vi "camera_diag.vi"() -> ()   [LabVIEW 2013]
uses:
  Program Files/Andor SOLIS/Drivers 32bit/Examples/LabVIEW/System Files/user.lib/atmcd32d.llb/AcquisitionMode_mode typedef.ctl
  Program Files/Andor SOLIS/Drivers 32bit/Examples/LabVIEW/System Files/user.lib/atmcd32d.llb/ReadMode_mode typedef.ctl
  Program Files/Andor SOLIS/Drivers 32bit/Examples/LabVIEW/System Files/user.lib/atmcd32d.llb/Error Code Enum typedef.ctl
panel:
  out "Status":u32
  out "DLL error code 3":u32
  out "output array":i32[][](graph)
  in  "FT Mode":enum16{"OFF", "ON"}(ring)
  out "DLL error code 2":u32
  out "DLL error code":u32
  out "SetKinError":u32
  out "Calculated Exposure Value":sgl format="%.2f"
  out "Calculated Kinetic Value":sgl format="%.2f"
  in  "Exposure Time (secs)":sgl format="%.2f"
  in  "Number of Kinetics":i32
  in  "Kinetic Cycle Time (s)":sgl format="%.2f"
  in  "Trigger":u32(ring) items=["Internal", "External"]
  in  "mode":T1=enum."Single Scan"
  in  "shutdown":bool
  in  "GO":bool
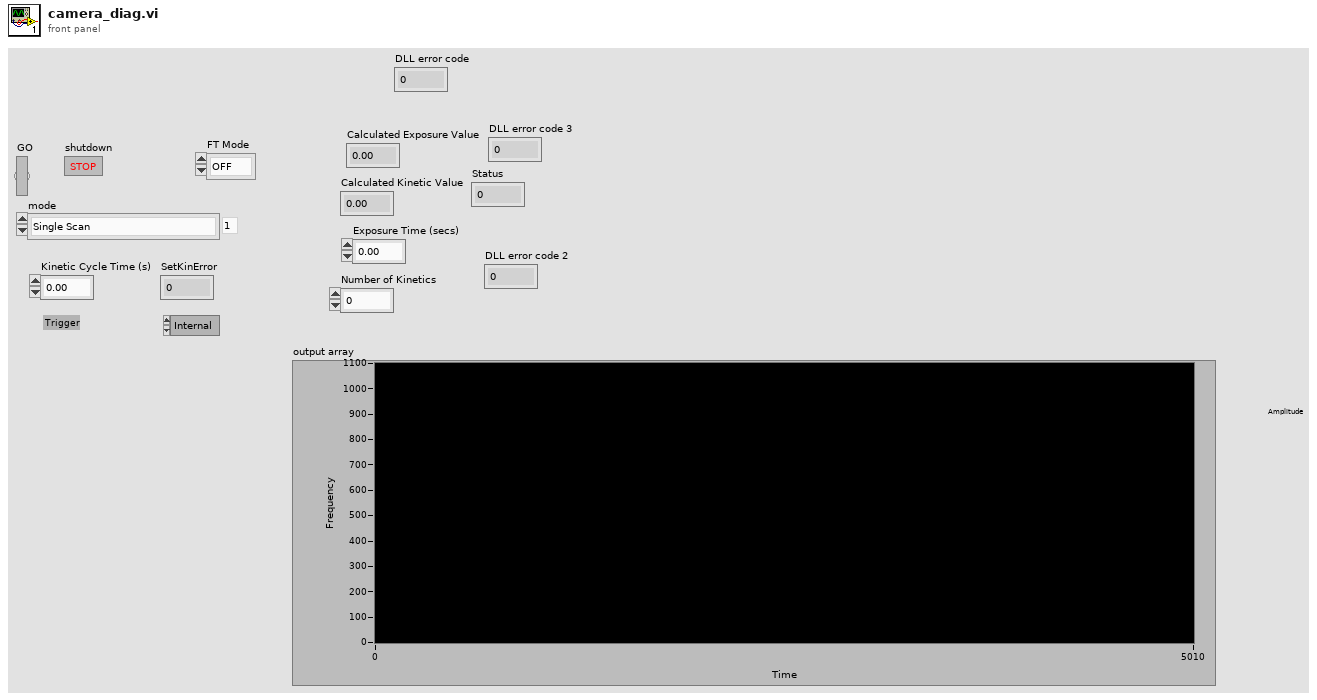
[diagram p1: front panel]
types:
  T1 = typedef "AcquisitionMode_mode typedef.ctl" = enum16{"Reserved (0)", "Single Scan", "Accumulate", "Kinetics", "Fast Kinetics", "Run Till Abort", "Reserved (6)", "Reserved (7)", "Reserved (8)", "Time Delayed Integration"}
  T2 = typedef "ReadMode_mode typedef.ctl" = enum16{"Full Vertical Binning", "Multi-Track", "Random-Track", "Single-Track", "Image"}
  T3 = typedef "Error Code Enum typedef.ctl" = enum32{"N/A (0)", "DRV_ERROR_CODES", "DRV_SUCCESS", "DRV_VXDNOTINSTALLED", "DRV_ERROR_SCAN", "DRV_ERROR_CHECK_SUM", "DRV_ERROR_FILELOAD", "DRV_UNKNOWN_FUNC", "DRV_ERROR_VXD_INIT", "DRV_ERROR_ADDRESS", "DRV_ERROR_PAGELOCK", "DRV_ERROR_PAGEUNLOCK", "DRV_ERROR_BOARDTEST", "DRV_ERROR_ACK", "DRV_ERROR_UP_FIFO", "DRV_ERROR_PATTERN", "N/A (16)", "DRV_ACQUISITION_ERRORS", "DRV_ACQ_BUFFER", "DRV_ACQ_DOWNFIFO_FULL", "DRV_PROC_UNKONWN_INSTRUCTION", "DRV_ILLEGAL_OP_CODE", "DRV_KINETIC_TIME_NOT_MET", "DRV_ACCUM_TIME_NOT_MET", "DRV_NO_NEW_DATA", "N/A (25)", "DRV_SPOOLERROR", "N/A (27)", "N/A (28)", "N/A (29)", "N/A (30)", "N/A (31)", "N/A (32)", "DRV_TEMPERATURE_CODES", "DRV_TEMPERATURE_OFF", "DRV_TEMPERATURE_NOT_STABILIZED", "DRV_TEMPERATURE_STABILIZED", "DRV_TEMPERATURE_NOT_REACHED", "DRV_TEMPERATURE_OUT_RANGE", "DRV_TEMPERATURE_NOT_SUPPORTED", "DRV_TEMPERATURE_DRIFT", "N/A (41)", "N/A (42)", "N/A (43)", "N/A (44)", "N/A (45)", "N/A (46)", "N/A (47)", "N/A (48)", "DRV_GENERAL_ERRORS", "DRV_INVALID_AUX", "DRV_COF_NOTLOADED", "DRV_FPGAPROG", "DRV_FLEXERROR", "DRV_GPIBERROR", "N/A (55)", "N/A (56)", "N/A (57)", "N/A (58)", "N/A (59)", "N/A (60)", "N/A (61)", "N/A (62)", "N/A (63)", "DRV_DATATYPE", "DRV_DRIVER_ERRORS", "DRV_P1INVALID", "DRV_P2INVALID", "DRV_P3INVALID", "DRV_P4INVALID", "DRV_INIERROR", "DRV_COFERROR", "DRV_ACQUIRING", "DRV_IDLE", "DRV_TEMPCYCLE", "DRV_NOT_INITIALIZED", "DRV_P5INVALID", "DRV_P6INVALID", "DRV_INVALID_MODE", "DRV_INVALID_FILTER", "DRV_I2CERRORS", "DRV_I2CDEVNOTFOUND", "DRV_I2CTIMEOUT", "DRV_P7INVALID", "N/A (84)", "N/A (85)", "N/A (86)", "N/A (87)", "N/A (88)", "N/A (89)", "DRV_IOCERROR", "DRV_VRMVERSIONERROR"}
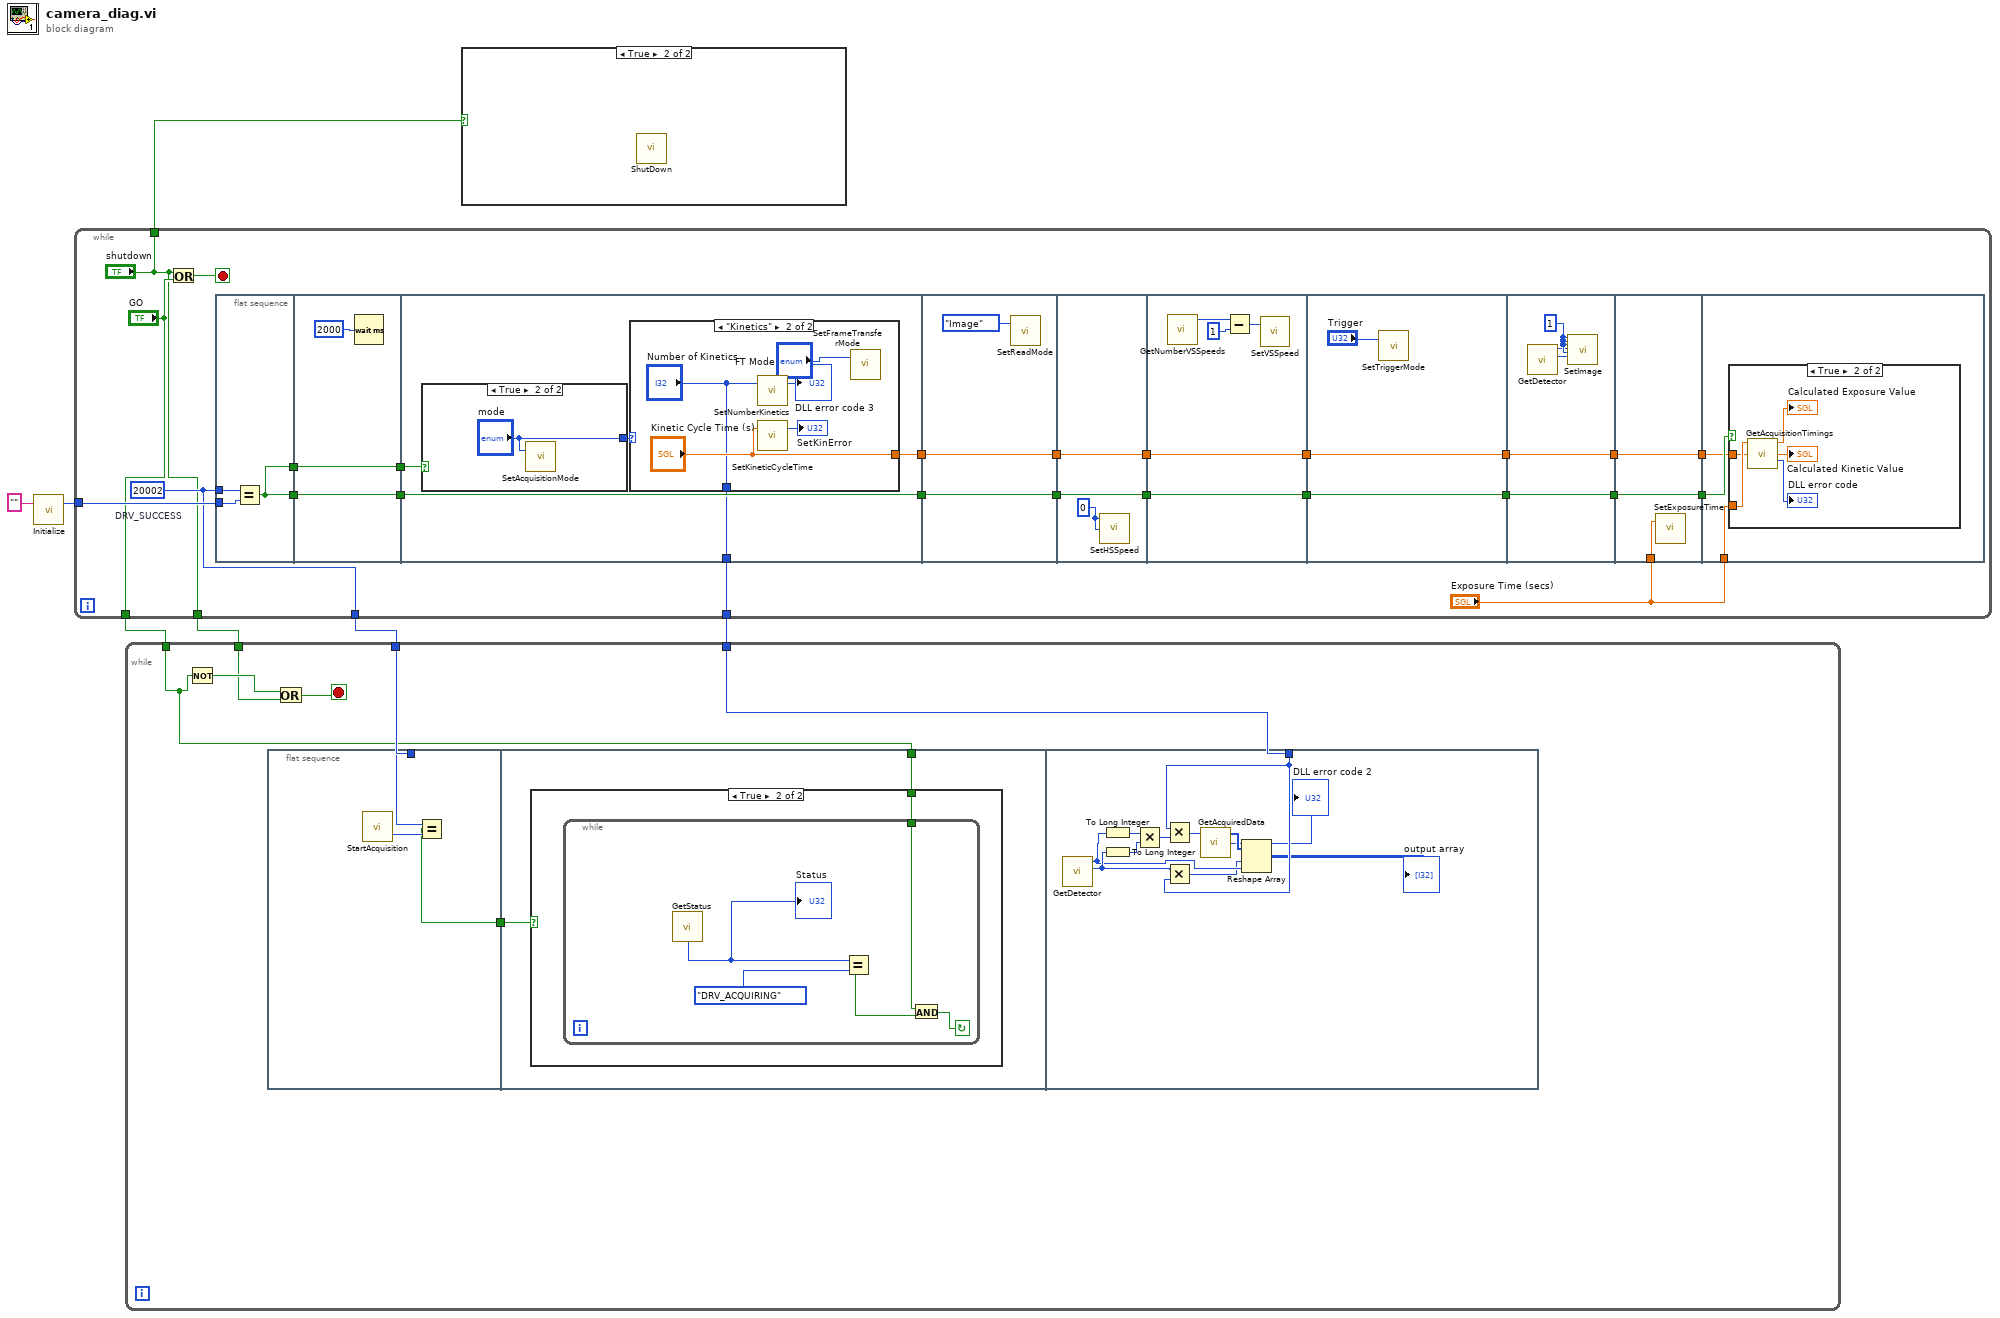
[diagram p0: block diagram]
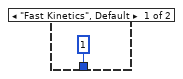
[diagram p4: hidden frame]
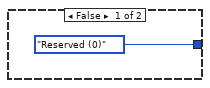
[diagram p5: hidden frame]
diagram:
  n1 = call "Initialize.vi"("directory (\"\")"="" ("directory (\"\")")) -> ("DLL error code"=w6:u32)  [unwired: 1 in, 1 out]
  n2 = while {
    tunnel: w6 -> [w31]
    tunnel: ["GO"] -> w5
    tunnel: [w10] -> w4
    tunnel: [w9] -> w3
    tunnel: ["shutdown"] -> w2
    tunnel: ["shutdown"] -> w1
    stop <- w32 stop-if-true
    w10 = 20002  # DRV_SUCCESS
    n3 = Or(x="shutdown", y="GO") -> (x .or. y?=w32:bool)
    n4 = flat-sequence {
      tunnel: w31 -> [w35]
      tunnel: w10 -> [w34]
      tunnel: [w33] -> w29
      tunnel: [w33] -> w20
      tunnel: [w37] -> w30
      tunnel: w29 -> [w37]
      tunnel: [w36] -> w21
      tunnel: w20 -> [w36]
      tunnel: w30 -> [w43]
      tunnel: [w41] -> w22
      tunnel: w21 -> [w41]
      tunnel: [w40] -> w12
      tunnel: [w39] -> w9
      tunnel: [w53] -> w23
      tunnel: w22 -> [w53]
      tunnel: [w52] -> w13
      tunnel: w12 -> [w52]
      tunnel: [w56] -> w24
      tunnel: w23 -> [w56]
      tunnel: [w55] -> w14
      tunnel: w13 -> [w55]
      tunnel: [w59] -> w25
      tunnel: w24 -> [w59]
      tunnel: [w58] -> w15
      tunnel: w14 -> [w58]
      tunnel: [w64] -> w26
      tunnel: w25 -> [w64]
      tunnel: [w63] -> w16
      tunnel: w15 -> [w63]
      tunnel: [w67] -> w27
      tunnel: w26 -> [w67]
      tunnel: [w66] -> w17
      tunnel: w16 -> [w66]
      tunnel: "Exposure Time (secs)" -> [w73]
      tunnel: [w72] -> w28
      tunnel: w27 -> [w72]
      tunnel: [w71] -> w18
      tunnel: w17 -> [w71]
      tunnel: w28 -> [w76]
      tunnel: "Exposure Time (secs)" -> [w75]
      tunnel: w18 -> [w74]
      frame #0 {
        n5 = Equal?(x=w34, y=w35) -> (x = y?=w33:bool)
      }
      frame #1 {
        n6 = Wait (ms)(milliseconds to wait=u32 2000) -> ()  [unwired: 1 out]
      }
      frame #2 {
        n7 = case shown="True" w43 {
          tunnel: [AcquisitionMode_mode_typedef."Reserved (0)" ("mode") "mode"] -> w42
          frame False {
          }
          frame True {
            n8 = call "SetAcquisitionMode.vi"("mode"="mode") -> ()  [unwired: 1 in, 2 out]
          }
        }
        n9 = case shown="\"Kinetics\"" w42 {
          tunnel: [_ "Kinetic Cycle Time (s)"] -> w40
          tunnel: [1 ("Number of Kinetics") "Number of Kinetics"] -> w39
          frame "Fast Kinetics", Default {
          }
          frame "Kinetics" {
            n10 = call <userlib>:"SetNumberKinetics.vi"("number"="Number of Kinetics") -> ("DLL error code"=→"DLL error code 3":u32)  [unwired: 1 in, 1 out]
            n11 = call <userlib>:"SetKineticCycleTime.vi"("time"="Kinetic Cycle Time (s)") -> ("DLL error code"=→"SetKinError":u32)  [unwired: 1 in, 1 out]
            n12 = call "SetFrameTransferMode.vi"("mode"="FT Mode") -> ()  [unwired: 1 in, 2 out]
          }
        }
      }
      frame #3 {
        n13 = call "SetReadMode.vi"("mode"=ReadMode_mode_typedef."Image") -> ()  [unwired: 1 in, 2 out]
      }
      frame #4 {
        w57 = 0
        n14 = call "SetHSSpeed.vi"("index"=w57, "type"=w57) -> ()  [unwired: 2 in, 2 out]
      }
      frame #5 {
        n15 = call "GetNumberVSSpeeds.vi"() -> ("number"=w62:i32)  [unwired: 3 in, 2 out]
        n16 = Subtract(x=w62, y=1) -> (x-y=w60:i32)
        n17 = call "SetVSSpeed.vi"("index"=w60) -> ()  [unwired: 1 in, 2 out]
      }
      frame #6 {
        n18 = call "SetTriggerMode.vi"("mode"="Trigger") -> ()  [unwired: 1 in, 2 out]
      }
      frame #7 {
        w70 = 1 ("hbin")
        n19 = call "GetDetector.vi"() -> ("ypixels"=w68:i32, "xpixels"=w69:i32)  [unwired: 4 in, 2 out]
        n20 = call "SetImage.vi"("hbin"=w70, "vbin"=w70, "hstart"=w70, "hend"=w69, "vstart"=w70, "vend"=w68) -> ()  [unwired: 20 in, 2 out]
      }
      frame #8 {
        n21 = call "SetExposureTime.vi"("time"=w73) -> ()  [unwired: 1 in, 2 out]
      }
      frame #9 {
        n22 = case shown="True" w76 {
          tunnel: w75 -> [_ w81]
          tunnel: w74 -> [_ w80]
          frame False {
          }
          frame True {
            n23 = call "GetAcquisitionTimings.vi"("exposure input"=w81, "kinetic input"=w80) -> ("exposure"=→"Calculated Exposure Value":sgl, "kinetic"=→"Calculated Kinetic Value":sgl, "DLL error code"=→"DLL error code":u32)  [unwired: 9 in, 2 out]
          }
        }
      }
    }
  }
  n24 = while {
    tunnel: w5 -> [w85]
    tunnel: w4 -> [w88]
    tunnel: w3 -> [w86]
    tunnel: w2 -> [w83]
    stop <- w82 stop-if-true
    n25 = Not(x=w85) -> (.not. x?=w84:bool)
    n26 = flat-sequence {
      tunnel: w88 -> [w90]
      tunnel: [w89] -> w87
      tunnel: w87 -> [w93]
      tunnel: w85 -> [w92]
      tunnel: w86 -> [w104]
      frame #0 {
        n27 = call "StartAcquisition.vi"() -> ("DLL error code"=w91:u32)  [unwired: 2 in, 1 out]
        n28 = Equal?(x=w90, y=w91) -> (x = y?=w89:bool)
      }
      frame #1 {
        n29 = case shown="True" w93 {
          tunnel: w92 -> [_ w94]
          frame False {
          }
          frame True {
            n30 = while {
              tunnel: w94 -> [w98]
              stop <- w96 continue-if-true
              n31 = call "GetStatus.vi"() -> ("status"=w95:T3)  [unwired: 3 in, 2 out]
              "Status" <- w95
              n32 = Equal?(x=w95, y=Error_Code_Enum_typedef."DRV_ACQUIRING") -> (x = y?=w97:bool)
              n33 = And(x=w98, y=w97) -> (x .and. y?=w96:bool)
            }
          }
        }
      }
      frame #2 {
        n34 = call "GetDetector.vi"() -> ("ypixels"=w105:i32, "xpixels"=w101:i32)  [unwired: 4 in, 2 out]
        n35 = To Long Integer(number=w101) -> (32bit integer=w110:i32)
        n36 = To Long Integer(number=w105) -> (32bit integer=w109:i32)
        n37 = Multiply(x=w110, y=w109) -> (x*y=w108:i32)
        n38 = Multiply(x=w104, y=w108) -> (x*y=w107:i32)
        n39 = Multiply(x=w105, y=w104) -> (x*y=w100:i32)
        n40 = call "GetAcquiredData.vi"("size"=w107) -> ("DLL error code"=→"DLL error code 2":u32, "array"=w106:i32[])  [unwired: 2 in, 1 out]
        n41 = Reshape Array(w106, w100, w101) -> (→"output array":i32[][])
      }
    }
    n42 = Or(x=w84, y=w83) -> (x .or. y?=w82:bool)
  }
  n43 = case shown="True" w1 {
    frame False {
    }
    frame True {
      n44 = call "ShutDown.vi"() -> ()  [unwired: 2 in, 2 out]
    }
  }
